vi "LineDecoder.vi"(8 "error in (no error)":errorcluster, 11 "Input Line":string) -> (0 "error out":errorcluster)   [LabVIEW 2018]
uses:
  <vilib>/Utility/Data Type/NI_Data Type.lvlib
panel:
  out "Array of Data":variant[](array[variant])
  in  "Data Types":variant[](array[variant])
  in  "Delimiters":string[](array[string])
  in  "Prompt":string
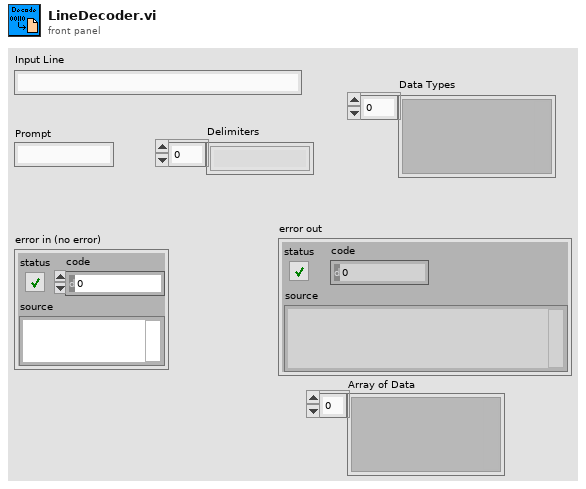
[diagram p1: front panel]
types:
  T1 = typedef "NI_Data Type.lvlib/Data Type.ctl" = enum8{"Invalid Type", "Void", "I8", "I16", "I32", "I64", "U8", "U16", "U32", "U64", "Single Float", "Double Float", "Extended Float", "Single Complex", "Double Complex", "Extended Complex", "Enum U8", "Enum U16", "Enum U32", "Enum U64", "Single Float With Unit", "Double Float With Unit", "Extended Float With Unit", "Single Complex with Unit", "Double Complex with Unit", "Extended Complex with Unit", "Boolean", "String", "Path", "Picture", "Tag", "Array", "Cluster", "Variant", "LV Variant", "Waveform", "Timestamp", "Digital Waveform", "Digital Data", "ExpressData", "Refnum", "External Data", "VI", "Poly VI", "LabVIEW Class Instance", "Fixed Point"}
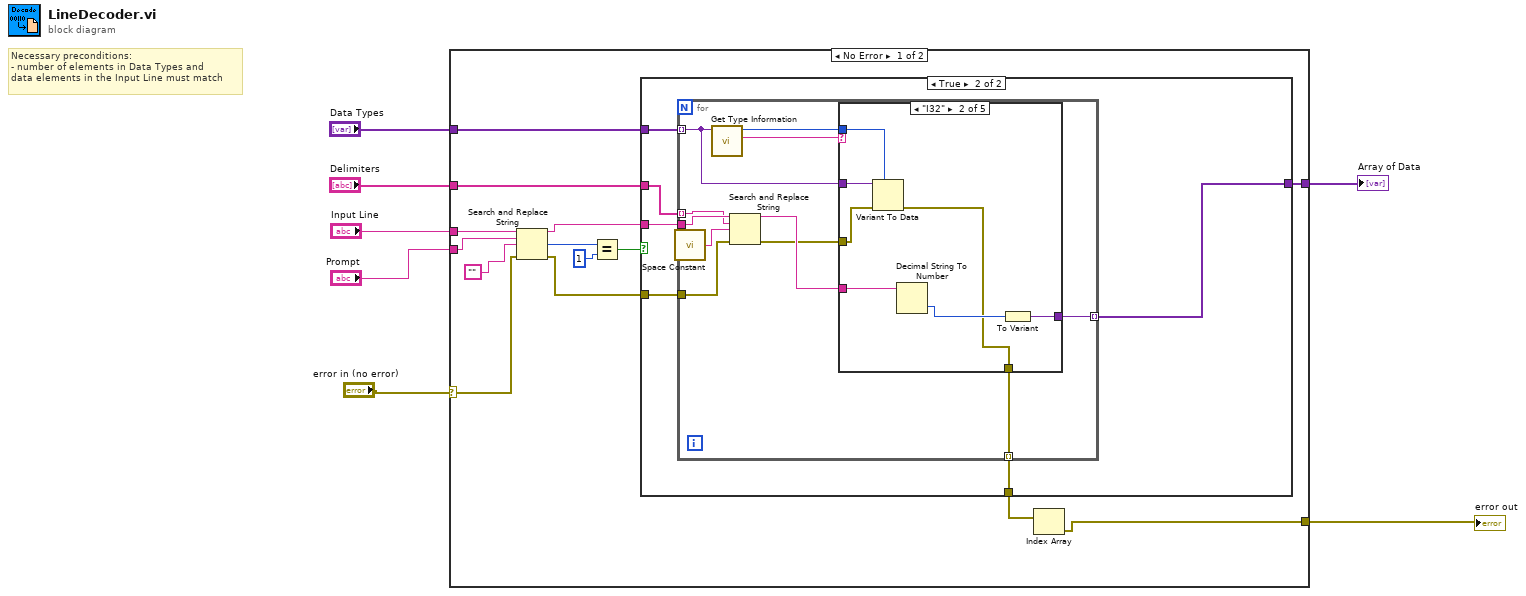
[diagram p0: block diagram]
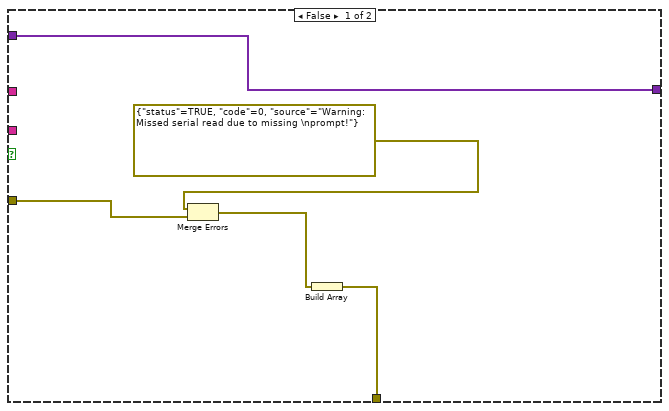
[diagram p2: hidden frame]
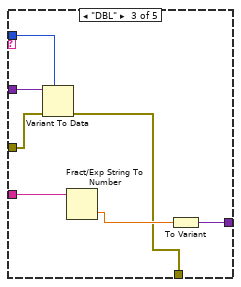
[diagram p4: hidden frame]
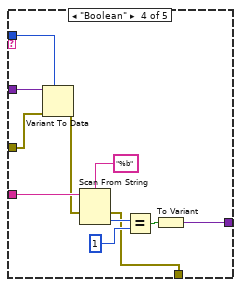
[diagram p5: hidden frame]
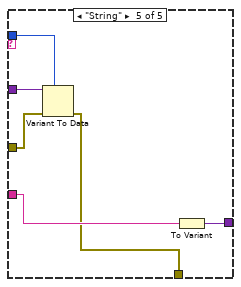
[diagram p6: hidden frame]
diagram:
  # "Necessary preconditions:\n- number of elements in Data Types and \ndata elements in the Input Line must match"
  n1 = case shown="No Error" "error in (no error)" {
    selector: "error in (no error)" -> [w20 w78]
    tunnel: "Input Line" -> [w21 _]
    tunnel: [w10 w78] -> w5
    tunnel: "Prompt" -> [w17 _]
    tunnel: "Delimiters" -> [w13 _]
    tunnel: "Data Types" -> [w12 w77]
    tunnel: [w11 w77] -> w1
    frame No Error {
      n2 = Search and Replace String(input string=w21, search string=w17, replace string="", error in=w20) -> (result string=w8:string, number of replacements=w16:i32, error out=w18:errorcluster)  [unwired: 4 in, 1 out]
      n3 = Equal?(x=w16, y=1) -> (x = y?=w14:bool)
      n4 = case shown="True" w14 {
        tunnel: w18 -> [w26 w29]
        tunnel: w13 -> [_ w31]
        tunnel: w12 -> [w22 w32]
        tunnel: [w22 w30] -> w11
        tunnel: [w23 w28] -> w9
        tunnel: w8 -> [_ w27]
        frame False {
          n5 = Merge Errors(errorcluster {"status"=TRUE, "code"=0, "source"="Warning: Missed serial read due to missing \nprompt!"} ("error constant"), w26) -> (w24:errorcluster)
          n6 = Build Array(w24) -> (w23:errorcluster[])
        }
        frame True {
          n7 = for {
            tunnel: w32 -> [w42] mode=indexing
            tunnel: w31 -> [w33] mode=indexing
            tunnel: [w39] -> w30 mode=indexing
            tunnel: w29 -> [w38]
            tunnel: [w36] -> w28 mode=indexing
            tunnel: w27 -> [w34]
            n8 = call <vilib>:"Space Constant.vi"() -> ("String"=w41:string)
            n9 = call <vilib>:"Get Type Information.vi"("Variant"=w42) -> ("Name"=w43:string, "Type"=w35:T1)  [unwired: 6 in, 3 out]
            n10 = Search and Replace String(input string=w34, search string=w33, replace string=w41, error in=w38) -> (result string=w40:string, error out=w37:errorcluster)  [unwired: 4 in, 2 out]
            n11 = case shown="\"I32\"" w43 {
              tunnel: w42 -> [w44 w52 w59 w70 w76]
              tunnel: w40 -> [_ w51 w58 w69 w74]
              tunnel: [w44 w50 w57 w64 w75] -> w39
              tunnel: w37 -> [w45 w48 w55 w63 w73]
              tunnel: [w45 w47 w54 w61 w72] -> w36
              tunnel: w35 -> [_ w46 w53 w60 w71]
              frame "Invalid Type", Default {
              }
              frame "I32" {
                n12 = Variant To Data(error in=w48, type=w46, Variant=w52) -> (error out=w47:errorcluster)  [unwired: 1 out]
                n13 = Decimal String To Number(string=w51) -> (number=w49:i32)  [unwired: 2 in, 1 out]
                n14 = To Variant(anything=w49) -> (Variant=w50:variant)
              }
              frame "DBL" {
                n15 = Variant To Data(error in=w55, type=w53, Variant=w59) -> (error out=w54:errorcluster)  [unwired: 1 out]
                n16 = Fract/Exp String To Number(string=w58) -> (number=w56:dbl)  [unwired: 3 in, 1 out]
                n17 = To Variant(anything=w56) -> (Variant=w57:variant)
              }
              frame "Boolean" {
                n18 = Variant To Data(error in=w63, type=w60, Variant=w70) -> (error out=w62:errorcluster)  [unwired: 1 out]
                n19 = Scan From String(format string="%b", input string=w69, error in=w62) -> (error out=w61:errorcluster, output 1=w67:i32)  [unwired: 2 in, 2 out]
                n20 = Equal?(x=w67, y=1) -> (x = y?=w65:bool)
                n21 = To Variant(anything=w65) -> (Variant=w64:variant)
              }
              frame "String" {
                n22 = Variant To Data(error in=w73, type=w71, Variant=w76) -> (error out=w72:errorcluster)  [unwired: 1 out]
                n23 = To Variant(anything=w74) -> (Variant=w75:variant)
              }
            }
          }
        }
      }
      n24 = Index Array(array=w9) -> (element=w10:errorcluster)  [unwired: 1 in]
    }
    frame Error {
    }
  }
  "error out" <- w5
  "Array of Data" <- w1
